vi "Create listbox text.vi"(8 "error in (no error)":errorcluster, 10 "ips available":string[](array[string]), 11 "Section Ref in":T1 format="%.0x") -> (0 "error out":errorcluster, 2 "listbox text":string[][](array[string]), 3 "Section Ref out":T1 format="%.0x", 5 "not present item indexes":i32[](array[numeric]))   [LabVIEW 2019]
uses:
  <vilib>/NI VeriStand/Custom Device API/Custom Device Item Ref.ctl
  <vilib>/NI VeriStand/Custom Device API/Get Item Property (String).vi
  ListboxGlobal.vi
  <vilib>/NI VeriStand/Custom Device API/Custom Device API.lvlib
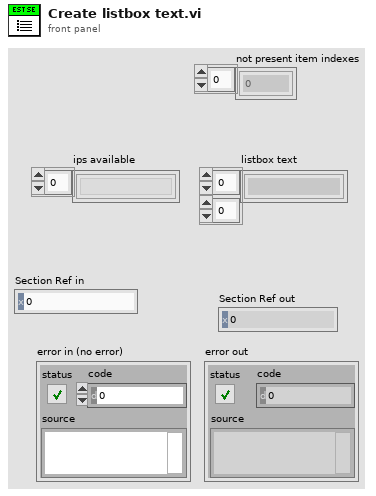
[diagram p1: front panel]
types:
  T1 = typedef "Custom Device API.lvlib/Custom Device Item Ref.ctl" = u64
  T2 = typedef "Custom Device API.lvlib/Custom Device Item Info.ctl" = cluster{"Name":string, "Is Channel":bool, "GUID":string, "Is Waveform":bool}
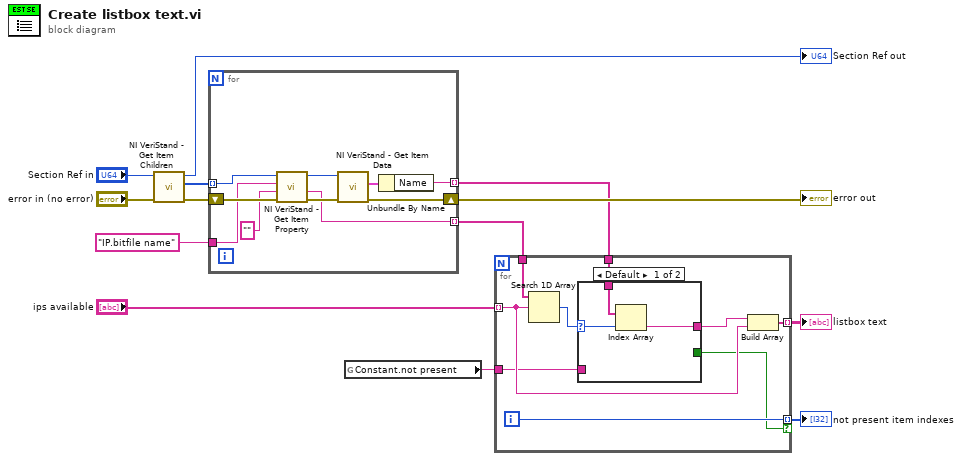
[diagram p0: block diagram]
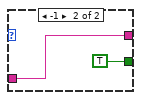
[diagram p2: hidden frame]
diagram:
  n1 = call <vilib>:"NI VeriStand - Get Item Children.vi"("error in (no error)"="error in (no error)", "Item Ref in"="Section Ref in") -> ("error out"=w11:errorcluster, "Child Refs"=w10:T1[], "Item Ref out"=→"Section Ref out":T1)  [unwired: 6 in, 1 out]
  n2 = for {
    shift-right: [w18] -> w8
    shift-left: w11 -> [w23]
    tunnel: w10 -> [w21] mode=indexing
    tunnel: "IP.bitfile name" ("IP.bitfile name") -> [w20]
    tunnel: [w15] -> w6 mode=indexing
    tunnel: [w14] -> w5 mode=indexing
    n3 = call-poly <vilib>:"NI VeriStand - Get Item Property.vi"("error in (no error)"=w23, "Default Value"="", "Property Name"=w20, "Item Ref in"=w21) -> ("error out"=w22:errorcluster, "Value"=w15:string, "Item Ref out"=w17:T1)  [unwired: 4 in, 1 out]
    n4 = call <vilib>:"NI VeriStand - Get Item Data.vi"("error in (no error)"=w22, "Item Ref in"=w17) -> ("error out"=w18:errorcluster, "Item Info"=w16:T2)  [unwired: 6 in, 2 out]
    n5 = Unbundle By Name(w16) -> ("Name"=w14:string)
  }
  "error out" <- w8
  n6 = global read "ListboxGlobal.vi" "Constant.not present"() -> (w2:string)
  n7 = for {
    tunnel: "ips available" -> [w28] mode=indexing
    tunnel: w6 -> [w32]
    tunnel: w5 -> [w30]
    tunnel: [w27] -> w4 mode=indexing
    tunnel: w2 -> [w26]
    tunnel: [w25] -> w3 mode=indexing if=w24
    i -> [w25]
    n8 = Search 1D Array(1D array=w32, element=w28) -> (index of element=w31:i32)  [unwired: 1 in]
    n9 = case shown="Default" w31 {
      selector: w31 -> [w34 _]
      tunnel: [w33 w37] -> w29
      tunnel: w30 -> [w35 _]
      tunnel: w26 -> [_ w37]
      tunnel: [_ TRUE] -> w24
      frame Default {
        n10 = Index Array(array=w35, index=w34) -> (element=w33:string)
      }
      frame -1 {
      }
    }
    n11 = Build Array(w29, w28) -> (w27:string[])
  }
  "listbox text" <- w4
  "not present item indexes" <- w3
